vi "test_TCP_2_RT.vi"() -> ()   [LabVIEW 2014]
panel:
  out "error out 2":errorcluster
  out "error out":errorcluster
  in  "stop":bool
  out "string":string
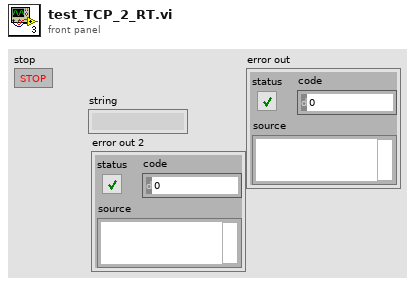
[diagram p1: front panel]
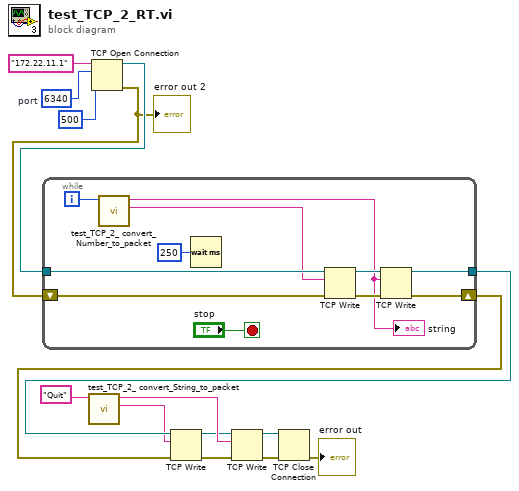
[diagram p0: block diagram]
diagram:
  w15 = u16 6340  # port
  n1 = call "test_TCP_2_ convert_String_to_packet.vi"("input_string"="Quit" ("data in")) -> ("output_PrePacket"=w1:string, "output_packet"=w6:string)  [unwired: 9 in]
  n2 = TCP Open Connection(address="172.22.11.1", remote port or service name=w15, timeout ms (60000)=500) -> (connection ID=w13:refnum<k5>, error out=w12:errorcluster)  [unwired: 2 in]
  "error out 2" <- w12
  n3 = while {
    tunnel: w13 -> [w21]
    shift-right: [w25] -> w2
    shift-left: w12 -> [w22]
    tunnel: [w24] -> w3
    i -> [w18]
    stop <- "stop" stop-if-true
    n4 = call "test_TCP_2_ convert_Number_to_packet.vi"("input_Number"=w18) -> ("output_PrePacket"=w16:string, "output_packet"=w17:string)  [unwired: 9 in]
    "string" <- w17
    n5 = Wait (ms)(milliseconds to wait=u32 250) -> ()  [unwired: 1 out]
    n6 = TCP Write(connection ID=w21, data in=w16, error in (no error)=w22) -> (connection ID out=w19:refnum<k5>, error out=w20:errorcluster)  [unwired: 1 in, 1 out]
    n7 = TCP Write(connection ID=w19, data in=w17, error in (no error)=w20) -> (connection ID out=w24:refnum<k5>, error out=w25:errorcluster)  [unwired: 2 out]
  }
  n8 = TCP Write(connection ID=w3, data in=w1, error in (no error)=w2) -> (connection ID out=w4:refnum<k5>, error out=w5:errorcluster)  [unwired: 2 out]
  n9 = TCP Write(connection ID=w4, data in=w6, error in (no error)=w5) -> (connection ID out=w10:refnum<k5>, error out=w11:errorcluster)  [unwired: 2 out]
  n10 = TCP Close Connection(connection ID=w10, error in (no error)=w11) -> (error out=→"error out":errorcluster)  [unwired: 1 in, 1 out]
